vi "Is Rect-Rect Collision.vi"(1 "Other Collider in":refnum<class "Rect Collider.lvclass">, 2 "Other object in":refnum<class "SimulationObject.lvclass">, 3 "Self Collider in":refnum<class "Rect Collider.lvclass">, 4 "Self Object in":refnum<class "SimulationObject.lvclass">) -> (0 "Are Colliding":bool)   [LabVIEW 2022 SP3, in "Rect Collider.lvclass"]
uses:
  Rect Collider.lvclass
  SimulationObject/SimulationObject.lvclass
  SimulationObject/SimulationObject.lvclass/SimulationObject.ctl
  Components/Transform/Transform.lvclass/Transform.ctl
  Math/Vector2/Vector2.lvclass/Vector2.ctl
  Rect Collider.lvclass/Rect Collider.ctl
  Read Width.vi
  Read Height.vi
  Math/Vector2/Read x.vi
  Math/Vector2/Read y.vi
  Components/Transform/Transform.lvclass
  Math/Vector2/Vector2.lvclass
  Shapes/RectangleShape/RectangleShape.lvclass
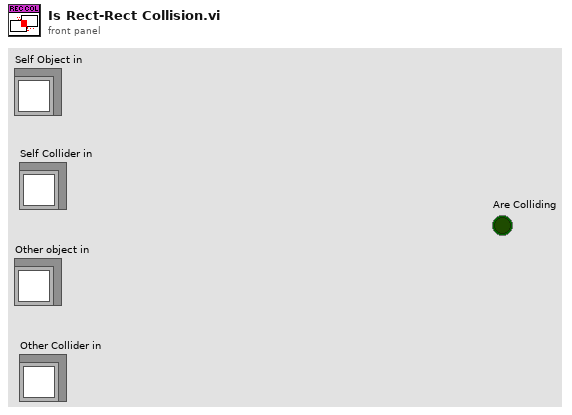
[diagram p1: front panel]
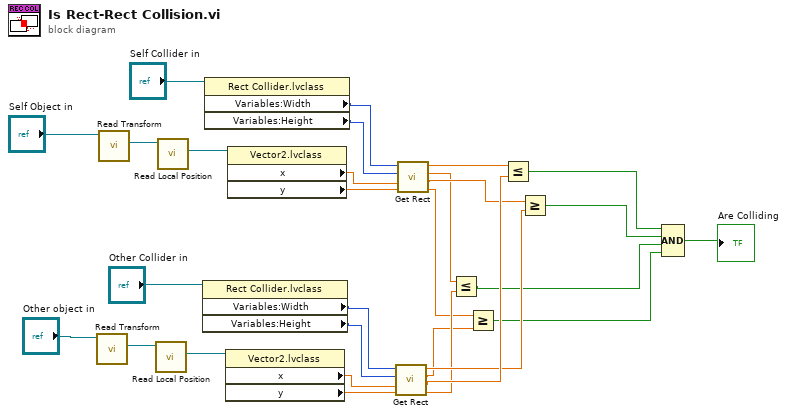
[diagram p0: block diagram]
diagram:
  n1 = call "Read Transform.vi"("SimulationObject in"="Other object in") -> ("Transform out"=w16:refnum<class "Transform.lvclass">)  [unwired: 8 in, 2 out]
  n2 = call "Read Transform.vi"("SimulationObject in"="Self Object in") -> ("Transform out"=w29:refnum<class "Transform.lvclass">)  [unwired: 8 in, 2 out]
  n3 = call "Read Local Position.vi"("Transform in"=w16) -> ("Local Position out"=w17:refnum<class "Vector2.lvclass">)  [unwired: 8 in, 2 out]
  n4 = call "Read Local Position.vi"("Transform in"=w29) -> ("Local Position out"=w26:refnum<class "Vector2.lvclass">)  [unwired: 8 in, 2 out]
  n5 = property class="Rect Collider.lvclass"(reference="Other Collider in") -> ("Variables:Width"=w21:i16, "Variables:Height"=w20:i16)  [unwired: 1 in, 2 out]
  n6 = property class="Rect Collider.lvclass"(reference="Self Collider in") -> ("Variables:Width"=w22:i16, "Variables:Height"=w23:i16)  [unwired: 1 in, 2 out]
  n7 = property class="Vector2.lvclass"(reference=w17) -> ("x"=w19:sgl, "y"=w18:sgl)  [unwired: 1 in, 2 out]
  n8 = property class="Vector2.lvclass"(reference=w26) -> ("x"=w24:sgl, "y"=w25:sgl)  [unwired: 1 in, 2 out]
  n9 = call "Get Rect.vi"("y"=w18, "x"=w19, "Height"=w20, "Width"=w21) -> ("Bottom"=w8:sgl, "Right"=w12:sgl, "Top"=w6:sgl, "Left"=w10:sgl)
  n10 = call "Get Rect.vi"("y"=w25, "x"=w24, "Height"=w23, "Width"=w22) -> ("Bottom"=w7:sgl, "Right"=w11:sgl, "Top"=w9:sgl, "Left"=w13:sgl)
  n11 = Less Or Equal?(x=w9, y=w8) -> (x <= y?=w2:bool)
  n12 = Greater Or Equal?(x=w7, y=w6) -> (x >= y?=w1:bool)
  n13 = Less Or Equal?(x=w13, y=w12) -> (x <= y?=w4:bool)
  n14 = Greater Or Equal?(x=w11, y=w10) -> (x >= y?=w3:bool)
  n15 = Compound Arithmetic op=AND(w4, w3, w2, w1) -> (→"Are Colliding":bool)
